vi "分布统计.vi"(2 "道数":i32, 3 "数组":dbl[](array[numeric])) -> (0 "分布谱":dbl[](graph), 1 "大小":i32)   [LabVIEW 2014]
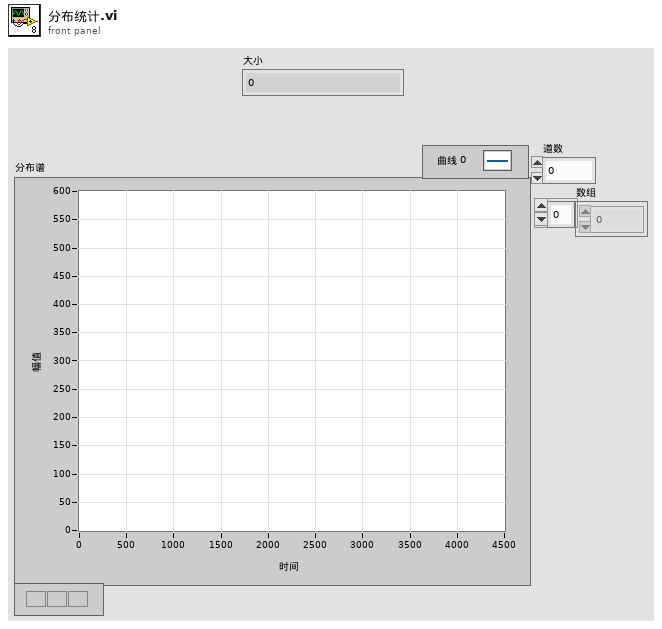
[diagram p1: front panel]
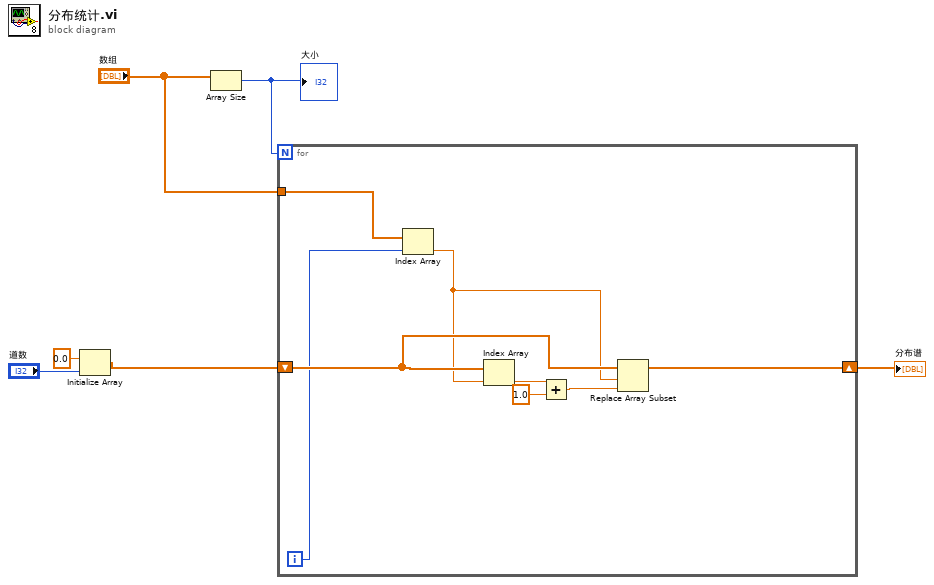
[diagram p0: block diagram]
diagram:
  n1 = Initialize Array(0.0 ("元素"), "道数") -> (w5:dbl[])
  n2 = Array Size(array="数组") -> (size(s)=w3:i32)
  "大小" <- w3
  n3 = for {
    N: w3 -> [_]
    tunnel: "数组" -> [w14]
    shift-right: [w12] -> w4
    shift-left: w5 -> [w13]
    i -> [w7]
    n4 = Index Array(array=w14, index=w7) -> (element=w9:dbl)
    n5 = Index Array(array=w13, index=w9) -> (element=w11:dbl)
    n6 = Add(x=w11, y=1.0) -> (x+y=w8:dbl)
    n7 = Replace Array Subset(array=w13, new element=w8, index=w9) -> (w12:dbl[])
  }
  "分布谱" <- w4
